vi "Dispense on kapton.vi"   [LabVIEW 2016]
uses:
  Workspace/Carrier Tray/Syringe Space/Syringe Space.lvclass
  Workspace/Carrier Tray/Assembly Tray.lvclass
  Secure Syringe/SecureRelease Syringe.lvclass
  Workspace/Pick Up Tool Area/Pick Up Tool.lvclass
  Pick and Place/Pick and Place Type.ctl
  Iterative Dispense/8 inch/8 inch Baseplate Dispense.lvclass
  8 inch Sensor Dispense.lvclass
  Pick and Place/Pick and Place.lvclass
  Workspace/Component/Component Tray.lvclass
  Pick and Place/Pick and Place.lvclass/Pick and Place.ctl
  Secure Syringe/SecureRelease Syringe.lvclass/SecureRelease Syringe.ctl
  Pick and Place/Write Pick and Place Type.vi
  Secure Syringe/Write Type.vi
  Controller/Controller.lvclass
types:
  T1 = typedef "Pick and Place.lvclass/Pick and Place Type.ctl" = enum16{"Primary Pick Up", "Secondary Pick Up", "Put Down All", "Pick Up All", "Put Down Secondary"}
  T2 = typedef "Controller.lvclass/Controllers.ctl" = cluster{"I-O.lvclass":refnum<class "I-O.lvclass">, "Motion.lvclass":refnum<class "Motion.lvclass">, "Dispenser.lvclass":refnum<class "Dispenser.lvclass">}
  T3 = typedef "Fixture.lvclass/Workspace.ctl" = cluster{"XYZTheta":dbl[], "Workspace Valve":i32, "Workspace Sensor":i32}
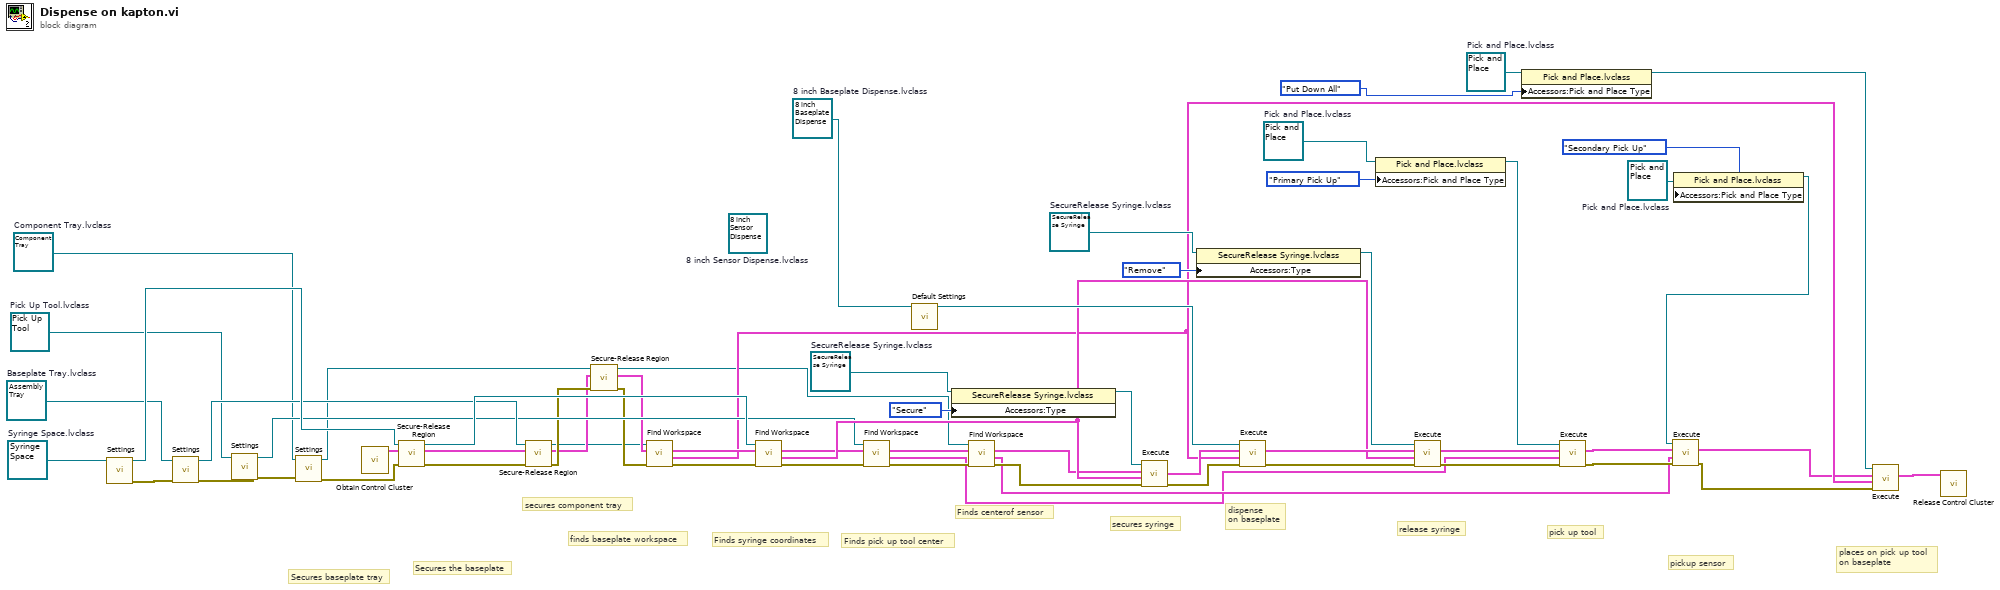
[diagram p0: block diagram]
diagram:
  w8 = refnum<class "Component Tray.lvclass"> refnum  # Component Tray.lvclass
  w23 = refnum<class "Pick and Place.lvclass"> refnum  # Pick and Place.lvclass
  (unwired) refnum<class "8 inch Sensor Dispense.lvclass"> refnum  # 8 inch Sensor Dispense.lvclass
  w25 = refnum<class "8 inch Baseplate Dispense.lvclass"> refnum  # 8 inch Baseplate Dispense.lvclass
  w35 = refnum<class "Pick and Place.lvclass"> refnum  # Pick and Place.lvclass
  w38 = refnum<class "Pick and Place.lvclass"> refnum  # Pick and Place.lvclass
  w43 = refnum<class "Pick Up Tool.lvclass"> refnum  # Pick Up Tool.lvclass
  w48 = refnum<class "SecureRelease Syringe.lvclass"> refnum  # SecureRelease Syringe.lvclass
  w56 = refnum<class "Assembly Tray.lvclass"> refnum  # Baseplate Tray.lvclass
  w59 = refnum<class "SecureRelease Syringe.lvclass"> refnum  # SecureRelease Syringe.lvclass
  w62 = refnum<class "Syringe Space.lvclass"> refnum  # Syringe Space.lvclass
  # "pickup sensor"
  # "Finds centerof sensor"
  # "Secures the baseplate"
  # "Secures baseplate tray"
  # "secures component tray"
  # "places on pick up tool\non baseplate"
  # "pick up tool"
  # "release syringe"
  # "dispense\non baseplate"
  # "secures syringe"
  # "Finds pick up tool center"
  # "Finds syringe coordinates"
  # "finds baseplate workspace"
  n1 = call-dynamic "Settings.vi"("Syringe Space in"=w62) -> ("error out"=w49:errorcluster, "Syringe Space out"=w61:refnum<class "Syringe Space.lvclass">)  [unwired: 9 in]
  n2 = call-dynamic "Settings.vi"("error in (no error)"=w49, "Baseplate Tray In"=w56) -> ("error out"=w42:errorcluster, "Baseplate Tray Out"=w55:refnum<class "Assembly Tray.lvclass">)  [unwired: 8 in]
  n3 = call-dynamic "Settings.vi"("error in (no error)"=w42, "Workspace in"=w43) -> ("error out"=w15:errorcluster, "Workspace out"=w41:refnum<class "Pick Up Tool.lvclass">)  [unwired: 8 in]
  n4 = call-dynamic "Settings.vi"("error in (no error)"=w15, "Component in"=w8) -> ("error out"=w14:errorcluster, "Component out"=w7:refnum<class "Component Tray.lvclass">)  [unwired: 8 in]
  n5 = call "Obtain Control Cluster.vi"() -> ("Control Out"=w54:T2)  [unwired: 11 in]
  n6 = call-dynamic "Secure-Release Region.vi"("error in (no error)"=w14, "Control In"=w54, "Baseplate Tray in"=w61) -> ("error out"=w31:errorcluster, "Control Out"=w53:T2, "Baseplate Tray out"=w60:refnum<class "Syringe Space.lvclass">)  [unwired: 6 in]
  n7 = call-dynamic "Secure-Release Region.vi"("error in (no error)"=w31, "Control In"=w53, "Baseplate Tray in"=w55) -> ("error out"=w12:errorcluster, "Control Out"=w10:T2, "Baseplate Tray out"=w1:refnum<class "Assembly Tray.lvclass">)  [unwired: 6 in]
  n8 = call-dynamic "Secure-Release Region.vi"("error in (no error)"=w12, "Control In"=w10, "Component in"=w7) -> ("error out"=w11:errorcluster, "Control Out"=w9:T2, "Component out"=w6:refnum<class "Component Tray.lvclass">)  [unwired: 6 in]
  n9 = call-dynamic "Find Workspace.vi"("Error In"=w11, "Control In"=w9, "Baseplate Tray in"=w1) -> ("Error Out"=w30:errorcluster, "Workspace"=w24:T3, "Control Out"=w52:T2)  [unwired: 5 in, 1 out]
  n10 = call-dynamic "Find Workspace.vi"("Error In"=w30, "Control In"=w52, "Baseplate Tray in"=w60) -> ("Error Out"=w29:errorcluster, "Workspace"=w44:T3, "Control Out"=w40:T2)  [unwired: 5 in, 1 out]
  n11 = call-dynamic "Find Workspace.vi"("Error In"=w29, "Control In"=w40, "Pick Up Tool In"=w41) -> ("Error Out"=w13:errorcluster, "Workspace Out"=w3:T3, "Control Out"=w16:T2)  [unwired: 5 in, 1 out]
  n12 = call-dynamic "Default Settings.vi"("C4 Dispense in 2"=w25) -> ("C4 Dispense out 2"=w51:refnum<class "8 inch Baseplate Dispense.lvclass">)  [unwired: 9 in, 1 out]
  n13 = property class="SecureRelease Syringe.lvclass"(reference=w59, "Accessors:Type"=enum16{"Secure", "Remove"}."Secure" ("Type")) -> (reference out=w57:refnum<class "SecureRelease Syringe.lvclass">)  [unwired: 1 in, 1 out]
  n14 = call-dynamic "Find Workspace.vi"("error in (no error)"=w13, "Control In"=w16, "Component.lvclass"=w6) -> ("error out"=w17:errorcluster, "Workspace"=w4:T3, "Control Out"=w5:T2)  [unwired: 5 in, 1 out]
  n15 = call-dynamic "Execute.vi"("error in (no error)"=w17, "Workspace"=w44, "Control In"=w5, "Secure Syringe in"=w57) -> ("error out"=w28:errorcluster, "Control Out"=w50:T2)  [unwired: 5 in, 1 out]
  n16 = property class="SecureRelease Syringe.lvclass"(reference=w48, "Accessors:Type"=enum16{"Secure", "Remove"}."Remove" ("Type")) -> (reference out=w46:refnum<class "SecureRelease Syringe.lvclass">)  [unwired: 1 in, 1 out]
  n17 = call-dynamic "Execute.vi"("Error In"=w28, "Workspace"=w24, "Control In"=w50, "Dispense in"=w51) -> ("Error Out"=w27:errorcluster, "Control Out"=w45:T2)  [unwired: 5 in, 1 out]
  n18 = property class="Pick and Place.lvclass"(reference=w38, "Accessors:Pick and Place Type"=Pick_and_Place_Type."Primary Pick Up" ("Pick and Place Type")) -> (reference out=w36:refnum<class "Pick and Place.lvclass">)  [unwired: 1 in, 1 out]
  n19 = call-dynamic "Execute.vi"("error in (no error)"=w27, "Workspace"=w44, "Control In"=w45, "Secure Syringe in"=w46) -> ("error out"=w26:errorcluster, "Control Out"=w39:T2)  [unwired: 5 in, 1 out]
  n20 = property class="Pick and Place.lvclass"(reference=w35, "Accessors:Pick and Place Type"=Pick_and_Place_Type."Put Down All" ("Pick and Place Type")) -> (reference out=w33:refnum<class "Pick and Place.lvclass">)  [unwired: 1 in, 1 out]
  n21 = call-dynamic "Execute.vi"("error in (no error)"=w26, "Workspace"=w3, "Control In"=w39, "Pick and Place in"=w36) -> ("error out"=w19:errorcluster, "Control Out"=w20:T2)  [unwired: 5 in, 1 out]
  n22 = property class="Pick and Place.lvclass"(reference=w23, "Accessors:Pick and Place Type"=Pick_and_Place_Type."Secondary Pick Up" ("Pick and Place Type")) -> (reference out=w21:refnum<class "Pick and Place.lvclass">)  [unwired: 1 in, 1 out]
  n23 = call-dynamic "Execute.vi"("error in (no error)"=w19, "Workspace"=w4, "Control In"=w20, "Pick and Place in"=w21) -> ("error out"=w18:errorcluster, "Control Out"=w2:T2)  [unwired: 5 in, 1 out]
  n24 = call-dynamic "Execute.vi"("error in (no error)"=w18, "Workspace"=w24, "Control In"=w2, "Pick and Place in"=w33) -> ("Control Out"=w32:T2)  [unwired: 5 in, 2 out]
  n25 = call "Release Control Cluster.vi"("output cluster"=w32) -> ()  [unwired: 11 in]
